vi "ArmNetwork.vi"(8 "error in (no error)":errorcluster) -> (0 "error out":errorcluster)   [LabVIEW 2020]
doc: "Network for Arm\n\nInputs:\n -- error in -- cluster\n\nOutputs:\n -- error in -- cluster"
uses:
  <vilib>/Rock Robotics/Network Tables/NT Write Number.vi
  ArmGlobal.vi
  <vilib>/Rock Robotics/Network Tables/NT Write Boolean.vi
  <vilib>/Rock Robotics/Network Tables/NT Write String.vi
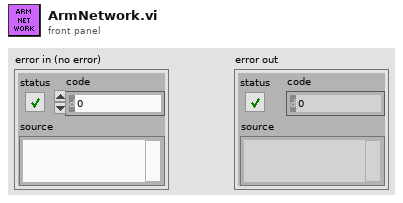
[diagram p1: front panel]
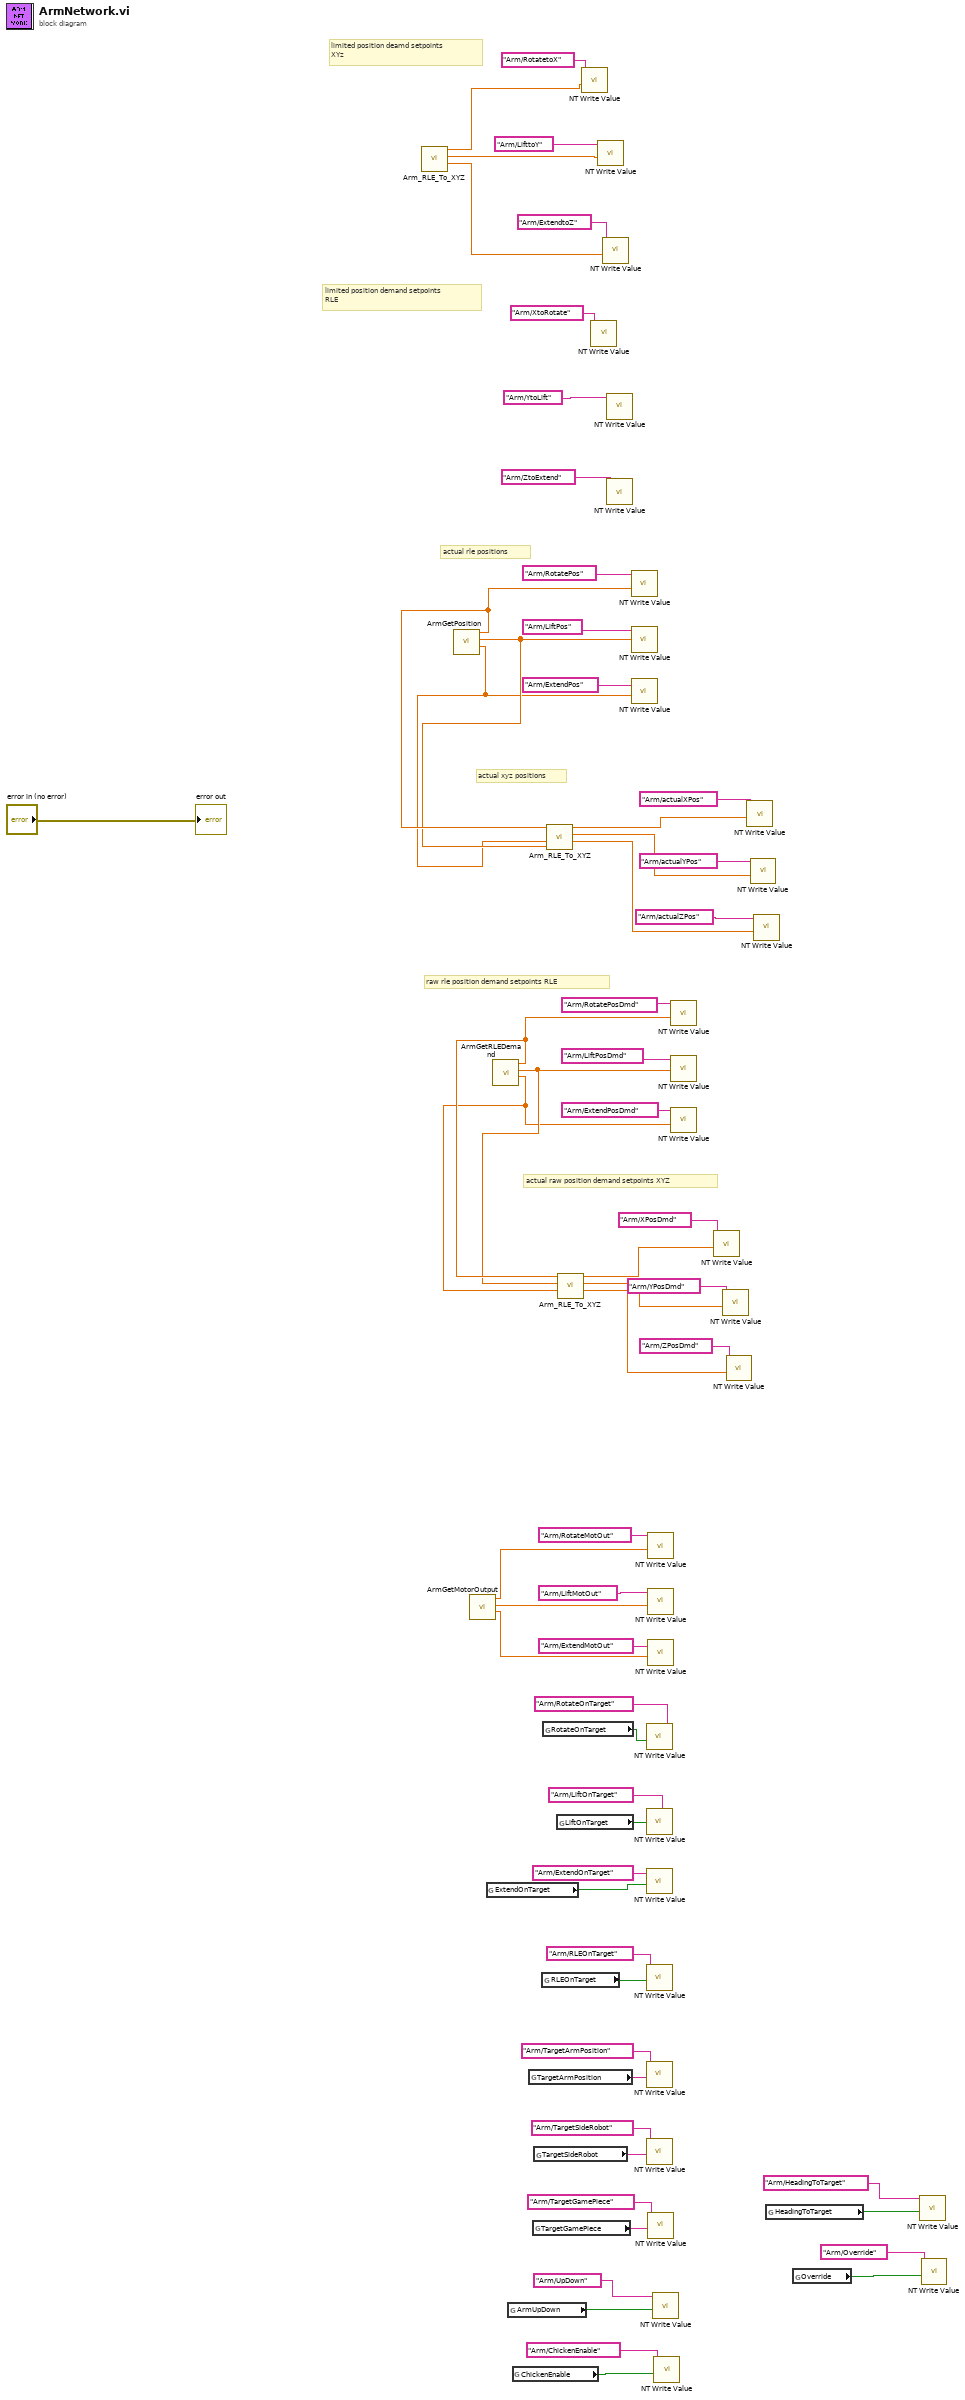
[diagram p0: block diagram]
diagram:
  # "actual xyz positions"
  # "actual raw position demand setpoints XYZ"
  # "limited position deamd setpoints\nXYz"
  # "limited position demand setpoints\nRLE"
  # "actual rle positions"
  # "raw rle position demand setpoints RLE"
  n1 = call "Arm_RLE_To_XYZ.vi"() -> ("z"=w23:dbl, "y"=w24:dbl, "x"=w25:dbl)  [unwired: 9 in]
  n2 = call "ArmGetPosition.vi"() -> ("ExtendPostion"=w14:dbl, "LiftPostion"=w21:dbl, "RotatePostion"=w22:dbl)  [unwired: 9 in]
  n3 = call "ArmGetMotorOutput.vi"() -> ("ExtendMotorOutput"=w59:dbl, "LiftMotorOutput"=w60:dbl, "RotateMotorOutput"=w61:dbl)  [unwired: 9 in]
  n4 = global read "ArmGlobal.vi" "ExtendOnTarget"() -> (w45:bool)
  n5 = call "ArmGetRLEDemand.vi"() -> ("ExtendPositonDemand(in)"=w11:dbl, "LiftPositionDemand(d)"=w12:dbl, "RotatePositonDemand(d)"=w13:dbl)  [unwired: 9 in]
  n6 = global read "ArmGlobal.vi" "ArmUpDown"() -> (w35:bool)
  n7 = global read "ArmGlobal.vi" "ChickenEnable"() -> (w33:bool)
  n8 = global read "ArmGlobal.vi" "TargetArmPosition"() -> (w41:string)
  n9 = global read "ArmGlobal.vi" "TargetGamePiece"() -> (w37:string)
  n10 = global read "ArmGlobal.vi" "TargetSideRobot"() -> (w39:string)
  n11 = global read "ArmGlobal.vi" "RLEOnTarget"() -> (w43:bool)
  n12 = global read "ArmGlobal.vi" "RotateOnTarget"() -> (w49:bool)
  n13 = call "Arm_RLE_To_XYZ.vi"("Extend"=w14, "Lift"=w21, "Rotate"=w22) -> ("z"=w18:dbl, "y"=w19:dbl, "x"=w20:dbl)  [unwired: 6 in]
  n14 = global read "ArmGlobal.vi" "LiftOnTarget"() -> (w48:bool)
  n15 = call "Arm_RLE_To_XYZ.vi"("Extend"=w11, "Lift"=w12, "Rotate"=w13) -> ("z"=w8:dbl, "y"=w9:dbl, "x"=w10:dbl)  [unwired: 6 in]
  n16 = call-poly <vilib>:"NT Write Value.vi"("value"=w25, "name"="Arm/RotatetoX") -> ()  [unwired: 9 in, 1 out]
  n17 = call-poly <vilib>:"NT Write Value.vi"("name"="Arm/XtoRotate") -> ()  [unwired: 10 in, 1 out]
  n18 = call-poly <vilib>:"NT Write Value.vi"("value"=w24, "name"="Arm/LifttoY") -> ()  [unwired: 9 in, 1 out]
  n19 = call-poly <vilib>:"NT Write Value.vi"("value"=w23, "name"="Arm/ExtendtoZ") -> ()  [unwired: 9 in, 1 out]
  n20 = call-poly <vilib>:"NT Write Value.vi"("name"="Arm/YtoLift") -> ()  [unwired: 10 in, 1 out]
  n21 = call-poly <vilib>:"NT Write Value.vi"("name"="Arm/ZtoExtend") -> ()  [unwired: 10 in, 1 out]
  n22 = call-poly <vilib>:"NT Write Value.vi"("value"=w22, "name"="Arm/RotatePos") -> ()  [unwired: 9 in, 1 out]
  n23 = call-poly <vilib>:"NT Write Value.vi"("value"=w21, "name"="Arm/LiftPos") -> ()  [unwired: 9 in, 1 out]
  n24 = call-poly <vilib>:"NT Write Value.vi"("value"=w14, "name"="Arm/ExtendPos") -> ()  [unwired: 9 in, 1 out]
  n25 = call-poly <vilib>:"NT Write Value.vi"("value"=w49, "name"="Arm/RotateOnTarget") -> ()  [unwired: 9 in, 1 out]
  n26 = call-poly <vilib>:"NT Write Value.vi"("value"=w48, "name"="Arm/LiftOnTarget") -> ()  [unwired: 9 in, 1 out]
  n27 = call-poly <vilib>:"NT Write Value.vi"("value"=w45, "name"="Arm/ExtendOnTarget") -> ()  [unwired: 9 in, 1 out]
  n28 = call-poly <vilib>:"NT Write Value.vi"("value"=w43, "name"="Arm/RLEOnTarget") -> ()  [unwired: 9 in, 1 out]
  n29 = call-poly <vilib>:"NT Write Value.vi"("value"=w41, "name"="Arm/TargetArmPosition") -> ()  [unwired: 9 in, 1 out]
  n30 = call-poly <vilib>:"NT Write Value.vi"("value"=w39, "name"="Arm/TargetSideRobot") -> ()  [unwired: 9 in, 1 out]
  n31 = call-poly <vilib>:"NT Write Value.vi"("value"=w61, "name"="Arm/RotateMotOut") -> ()  [unwired: 9 in, 1 out]
  n32 = call-poly <vilib>:"NT Write Value.vi"("value"=w60, "name"="Arm/LiftMotOut") -> ()  [unwired: 9 in, 1 out]
  n33 = call-poly <vilib>:"NT Write Value.vi"("value"=w59, "name"="Arm/ExtendMotOut") -> ()  [unwired: 9 in, 1 out]
  n34 = call-poly <vilib>:"NT Write Value.vi"("value"=w37, "name"="Arm/TargetGamePiece") -> ()  [unwired: 9 in, 1 out]
  n35 = call-poly <vilib>:"NT Write Value.vi"("value"=w35, "name"="Arm/UpDown") -> ()  [unwired: 9 in, 1 out]
  n36 = call-poly <vilib>:"NT Write Value.vi"("value"=w33, "name"="Arm/ChickenEnable") -> ()  [unwired: 9 in, 1 out]
  n37 = call-poly <vilib>:"NT Write Value.vi"("value"=w13, "name"="Arm/RotatePosDmd") -> ()  [unwired: 9 in, 1 out]
  n38 = call-poly <vilib>:"NT Write Value.vi"("value"=w12, "name"="Arm/LiftPosDmd") -> ()  [unwired: 9 in, 1 out]
  n39 = call-poly <vilib>:"NT Write Value.vi"("value"=w11, "name"="Arm/ExtendPosDmd") -> ()  [unwired: 9 in, 1 out]
  n40 = call-poly <vilib>:"NT Write Value.vi"("value"=w10, "name"="Arm/XPosDmd") -> ()  [unwired: 9 in, 1 out]
  n41 = call-poly <vilib>:"NT Write Value.vi"("value"=w9, "name"="Arm/YPosDmd") -> ()  [unwired: 9 in, 1 out]
  n42 = call-poly <vilib>:"NT Write Value.vi"("value"=w8, "name"="Arm/ZPosDmd") -> ()  [unwired: 9 in, 1 out]
  n43 = call-poly <vilib>:"NT Write Value.vi"("value"=w20, "name"="Arm/actualXPos") -> ()  [unwired: 9 in, 1 out]
  n44 = call-poly <vilib>:"NT Write Value.vi"("value"=w19, "name"="Arm/actualYPos") -> ()  [unwired: 9 in, 1 out]
  n45 = call-poly <vilib>:"NT Write Value.vi"("value"=w18, "name"="Arm/actualZPos") -> ()  [unwired: 9 in, 1 out]
  n46 = global read "ArmGlobal.vi" "HeadingToTarget"() -> (w4:bool)
  n47 = global read "ArmGlobal.vi" "Override"() -> (w2:bool)
  n48 = call-poly <vilib>:"NT Write Value.vi"("value"=w4, "name"="Arm/HeadingToTarget") -> ()  [unwired: 9 in, 1 out]
  n49 = call-poly <vilib>:"NT Write Value.vi"("value"=w2, "name"="Arm/Override") -> ()  [unwired: 9 in, 1 out]
  "error out" <- "error in (no error)"
